vi "Write to PGSQL.vi"(8 "error in (no error)":errorcluster, 9 "Variant":variant, 10 "Path":refnum<k21>, 11 "Logger in":refnum<class "Logger.PGSQL.lvclass">) -> (0 "error out":errorcluster, 3 "Logger out":refnum<class "Logger.PGSQL.lvclass">)   [LabVIEW 2016, in "Logger.PGSQL.lvclass"]
doc: "- If \"Variant\" is double, string, boolean, etc, \"Path\" should be the full path to the trace.\n- If \"Variant\" is a cluster, \"Path\" can just be the Process name. This VI will parse the cluster and write each element to its own trace. The name of each element must match the name of a trace in the DSC database."
uses:
  Logger.PGSQL.lvclass
  <vilib>/Utility/Data Type/NI_Data Type.lvlib
  <vilib>/JKI/JKI SMO/URI Parsing/URI.lvlib
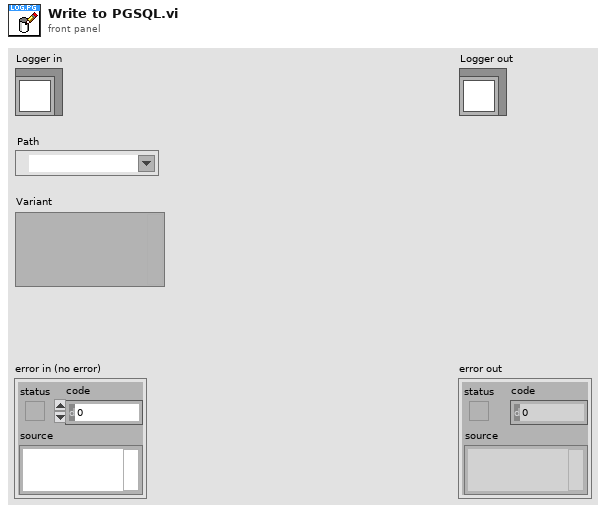
[diagram p1: front panel]
types:
  T1 = typedef "NI_Data Type.lvlib/Data Type.ctl" = enum8{"Invalid Type", "Void", "I8", "I16", "I32", "I64", "U8", "U16", "U32", "U64", "Single Float", "Double Float", "Extended Float", "Single Complex", "Double Complex", "Extended Complex", "Enum U8", "Enum U16", "Enum U32", "Enum U64", "Single Float With Unit", "Double Float With Unit", "Extended Float With Unit", "Single Complex with Unit", "Double Complex with Unit", "Extended Complex with Unit", "Boolean", "String", "Path", "Picture", "Tag", "Array", "Cluster", "Variant", "LV Variant", "Waveform", "Timestamp", "Digital Waveform", "Digital Data", "ExpressData", "Refnum", "External Data", "VI", "Poly VI", "LabVIEW Class Instance", "Fixed Point"}
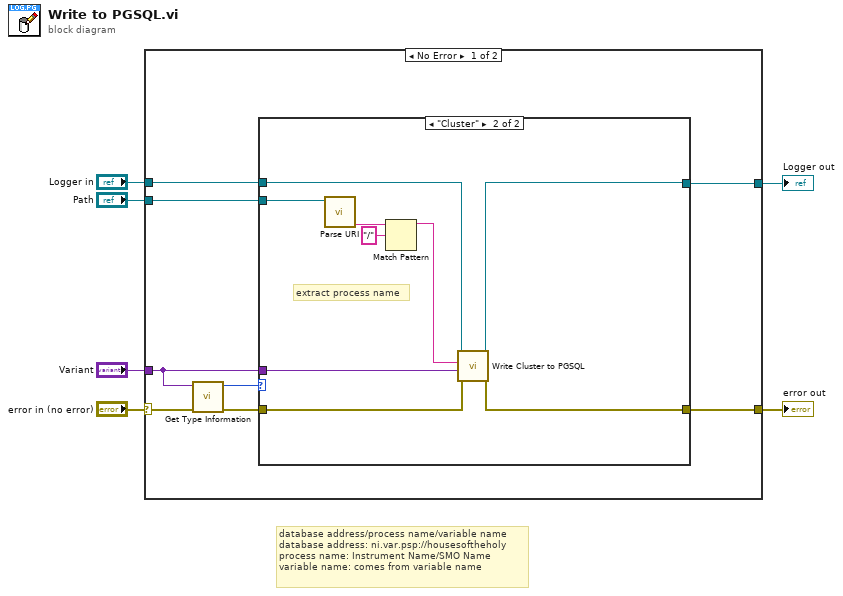
[diagram p0: block diagram]
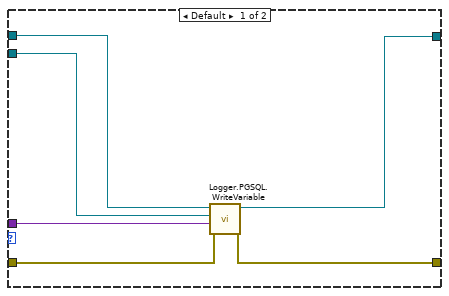
[diagram p2: hidden frame]
diagram:
  # "database address/process name/variable name\ndatabase address: ni.var.psp://housesoftheholy\nprocess name: Instrument Name/SMO Name\nvariable name: comes from variable name"
  n1 = case shown="No Error" "error in (no error)" {
    selector: "error in (no error)" -> [w11 w31]
    tunnel: [w8 w31] -> w5
    tunnel: [w7 w30] -> w3
    tunnel: "Logger in" -> [w9 w30]
    tunnel: "Variant" -> [w13 _]
    tunnel: "Path" -> [w10 _]
    frame No Error {
      n2 = call <vilib>:"Get Type Information.vi"("error in (no error)"=w11, "Variant"=w13) -> ("error out"=w12:errorcluster, "Type"=w14:T1)  [unwired: 5 in, 3 out]
      n3 = case shown="\"Cluster\"" w14 {
        tunnel: w10 -> [w20 w26]
        tunnel: [w15 w22] -> w8
        tunnel: w13 -> [w19 w29]
        tunnel: w12 -> [w16 w23]
        tunnel: w9 -> [w18 w28]
        tunnel: [w17 w27] -> w7
        frame Default {
          n4 = call "Logger.PGSQL.WriteVariable.vi"("error in (no error)"=w16, "Data"=w19, "Address"=w20, "Logger"=w18) -> ("error out"=w15:errorcluster, "Logger out"=w17:refnum<class "Logger.PGSQL.lvclass">)  [unwired: 6 in]
        }
        frame "Cluster" {
          # "extract process name"
          n5 = call <vilib>:"Parse URI.vi"("URI"=w26) -> ("path"=w21:string)  [unwired: 6 in, 4 out]
          n6 = Match Pattern(string=w21, regular expression="/") -> (before substring=w24:string)  [unwired: 1 in, 3 out]
          n7 = call-dynamic "Write Cluster to PGSQL.vi"("error in (no error)"=w23, "Variant"=w29, "Process name"=w24, "Logger in"=w28) -> ("error out"=w22:errorcluster, "Logger out"=w27:refnum<class "Logger.PGSQL.lvclass">)  [unwired: 6 in]
        }
      }
    }
    frame Error {
    }
  }
  "error out" <- w5
  "Logger out" <- w3
